vi "INIFilePath.vi"(8 "error in":errorcluster, 11 "ModisEdgeScanner.ini Filename":string="modisEdgeScanner.ini") -> (0 "error out":errorcluster, 3 "appended path":path)   [LabVIEW 2015]
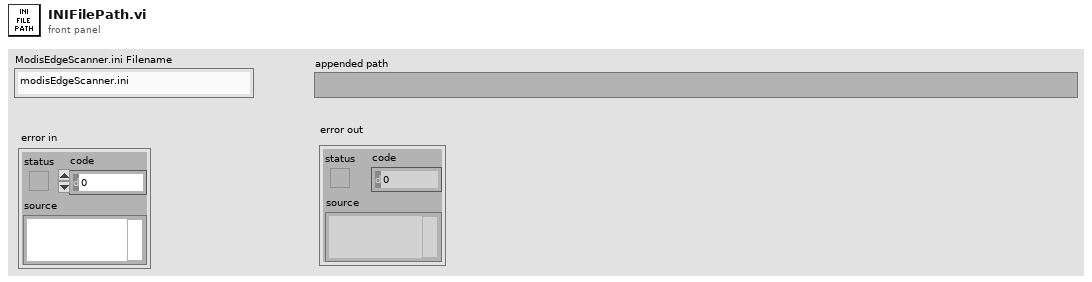
[diagram p1: front panel]
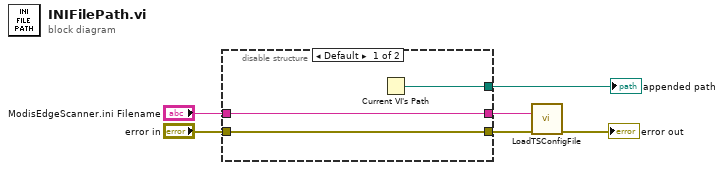
[diagram p0: block diagram]
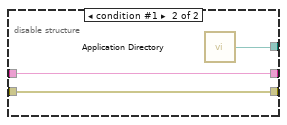
[diagram p2: hidden frame]
diagram:
  n1 = disable-structure shown="Default" {
    disable-tunnel: "ModisEdgeScanner.ini Filename" -> [w9 w11]
    disable-tunnel: [w7 w10] -> w5
    disable-tunnel: "error in" -> [w8 w12]
    disable-tunnel: [_ w12] -> w3
    disable-tunnel: [w9 w11] -> w2
    disable-tunnel: [w8 _] -> w1
    frame condition #0 (active) {
      n2 = Current VI's Path() -> (path=w7:path)
    }
    frame condition #1 {
      n3 = call <vilib>:"Application Directory.vi"() -> ("Application Directory"=w10:path)
    }
  }
  "error out" <- w3
  "appended path" <- w5
  n4 = call "LoadTSConfigFile.vi"("file name"=w2, "error in (no error)"=w1) -> ()  [unwired: 3 in, 11 out]
